vi "ProdaNG.ProcessResult.New.vi"(8 "error in (no error)":errorcluster, 10 "ProcessResult":T1, 11 "dbHandle":i32) -> (0 "error out":errorcluster, 2 "ProcessResult out":T1, 3 "dbHandle":i32)   [LabVIEW 2016]
doc: "This function creates a new Process result out of a prefilled process result structure.\nParameter:\nhandle is an Integer, which is returned by the function Login() at the creation of a new connection.\nprocessResult is a pointer on a process result structure, which elements must be prefilled. The structure must be defined and filled in the calling program. Nearly all elements of the structure must be set to reasonable values. The element id is filled by the DLL with a new Id for the created record, if the returncode is 0. The element startTime is filled automatically with the current time by the DLL and the endTime is deleted.\nThe element statusId is of particular importance:\nIf this element is passed with the value -1, the DLL automatically sets the standard value 2 (in Process), while otherwise the returned status is set.\nIn case of the returncode ERROR_MORE_DATA, the existing record is returned unchanged.\n\nReturncodes:\n0 No error\n234 (ERROR_MORE_DATA) in case, that the process result already exists for the process and the product. This is no error and the ProcessResult structure is returned with the existing result. \n< 0 ORACLE Error code\n 6 (ERROR_INVALID_HANDLE) in case of an invalid handle"
uses:
  Controls/ProdaNG.ProcessResult.ctl
  Controls/ProdaNG.ProcessResultSize.ctl
  prodllNG.dll
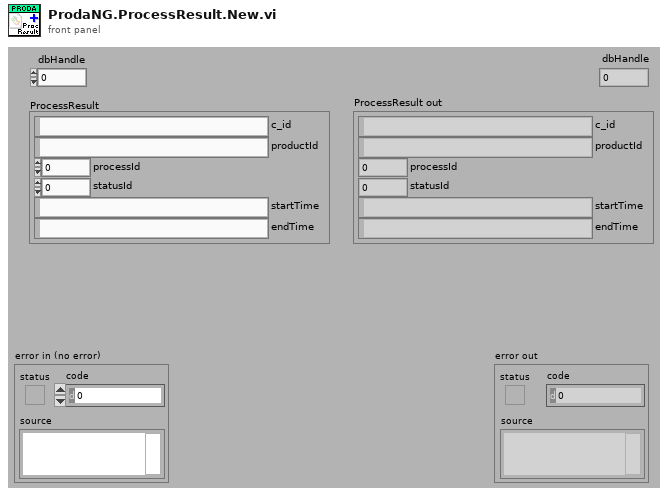
[diagram p1: front panel]
types:
  T1 = typedef "ProdaNG.ProcessResult.ctl" = cluster{"c_id":string, "productId":string, "processId":i32, "statusId":i32, "startTime":string, "endTime":string}
  T2 = typedef "ProdaNG.ProcessResultSize.ctl" = cluster{"c_id":i32, "productId":i32, "processId":i32, "statusId":i32, "startTime":i32, "endTime":i32}
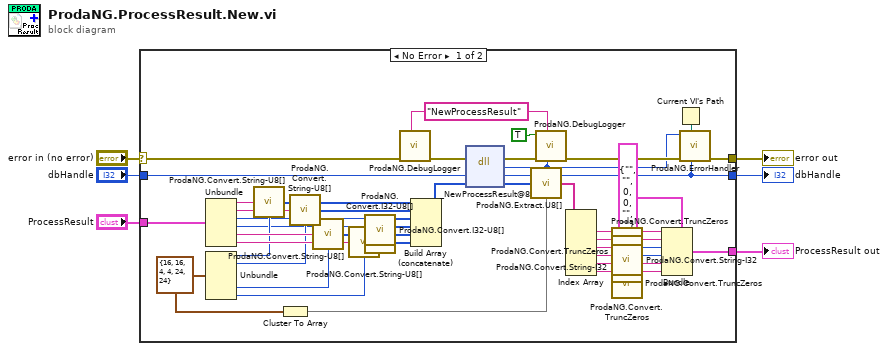
[diagram p0: block diagram]
diagram:
  n1 = case shown="No Error" "error in (no error)" {
    selector: "error in (no error)" -> [w38 w55]
    tunnel: [w49 w55] -> w5
    tunnel: [w22 _] -> w4
    tunnel: [w47 w54] -> w3
    tunnel: "ProcessResult" -> [w46 _]
    tunnel: "dbHandle" -> [w45 w54]
    frame No Error {
      w8 = T2 {"c_id"=16, "productId"=16, "processId"=4, "statusId"=4, "startTime"=24, "endTime"=24} ("ProcessResultSize")
      w44 = "NewProcessResult" ("cmd")
      n2 = Unbundle(w46) -> ("c_id"=w52:string, "productId"=w53:string, "processId"=w16:i32, "statusId"=w15:i32, "startTime"=w50:string, "endTime"=w51:string)
      n3 = Unbundle(w8) -> ("c_id"=w20:i32, "productId"=w18:i32, "startTime"=w9:i32, "endTime"=w10:i32)  [unwired: 2 out]
      n4 = call "ProdaNG.Convert.String-U8[].vi"("Input String"=w52, "Size"=w20) -> ("Output"=w19:u8[])
      n5 = Cluster To Array(cluster=w8) -> (array=w36:i32[])
      n6 = call "ProdaNG.Convert.String-U8[].vi"("Input String"=w53, "Size"=w18) -> ("Output"=w17:u8[])
      n7 = call "ProdaNG.Convert.String-U8[].vi"("Input String"=w50, "Size"=w9) -> ("Output"=w11:u8[])
      n8 = call "ProdaNG.Convert.String-U8[].vi"("Input String"=w51, "Size"=w10) -> ("Output"=w12:u8[])
      n9 = call "ProdaNG.Convert.I32-U8[].vi"("32bit integer"=w16) -> ("unsigned byte array"=w14:u8[])  [unwired: 10 in]
      n10 = call "ProdaNG.Convert.I32-U8[].vi"("32bit integer"=w15) -> ("unsigned byte array"=w13:u8[])  [unwired: 10 in]
      n11 = call "ProdaNG.DebugLogger.vi"("cmd"=w44, "error in (no error)"=w38) -> ("error out"=w39:errorcluster)  [unwired: 9 in]
      n12 = Build Array (concatenate)(w19, w17, w14, w13, w11, w12) -> (w7:u8[])
      n13 = dll-call lib="D:/Maszup/WABCO/SVN/LineTraceSystem/SOFTWARE/sources/Database/ProdaNG/prodllNG.dll" fn="_NewProcessResult@8" ("ProDll.dll:InitProDll")(error in=w39, "dbHandle"=w45, "processResult"=w7) -> (error out=w42:errorcluster, "return type"=w40:i32, "dbHandle"=w47:i32, "processResult"=w21:u8[])  [unwired: 2 in, 1 out]
      n14 = call "ProdaNG.Extract.U8[].vi"("unsigned byte array"=w21, "Sizes"=w36) -> ("Elements"=w37:string[])
      n15 = call "ProdaNG.DebugLogger.vi"("return type"=w40, "cmd"=w44, "error in (no error)"=w42, "done? (F)"=TRUE) -> ("error out"=w41:errorcluster)  [unwired: 7 in]
      n16 = Index Array(array=w37) -> (element #1=w24:string, element #2=w23:string, element #3=w34:string, element #4=w31:string, element #5=w28:string, element #6=w30:string)  [unwired: 6 in]
      n17 = call "ProdaNG.Convert.TruncZeros.vi"("string with \\0s"=w24) -> ("LV string"=w26:string)  [unwired: 10 in]
      n18 = call "ProdaNG.Convert.TruncZeros.vi"("string with \\0s"=w23) -> ("LV string"=w25:string)  [unwired: 10 in]
      n19 = call "ProdaNG.Convert.String-I32.vi"("unsigned byte string"=w34) -> ("32bit integer"=w33:i32)  [unwired: 10 in]
      n20 = call "ProdaNG.Convert.String-I32.vi"("unsigned byte string"=w31) -> ("32bit integer"=w32:i32)  [unwired: 10 in]
      n21 = call "ProdaNG.Convert.TruncZeros.vi"("string with \\0s"=w28) -> ("LV string"=w27:string)  [unwired: 10 in]
      n22 = call "ProdaNG.Convert.TruncZeros.vi"("string with \\0s"=w30) -> ("LV string"=w29:string)  [unwired: 10 in]
      n23 = Bundle(cluster=T1 {"c_id"="", "productId"="", "processId"=0, "statusId"=0, "startTime"="", "endTime"=""} ("ProcessResult"), "c_id"=w26, "productId"=w25, "processId"=w33, "statusId"=w32, "startTime"=w27, "endTime"=w29) -> (w22:T1)
      n24 = Current VI's Path() -> (path=w48:path)
      n25 = call "ProdaNG.ErrorHandler.vi"("dbHandleIn"=w47, "Path"=w48, "error in"=w41, "output_parameter"=w40) -> ("error out"=w49:errorcluster)  [unwired: 7 in]
    }
    frame Error {
    }
  }
  "error out" <- w5
  "ProcessResult out" <- w4
  "dbHandle" <- w3
